vi "Acquire Image.vi"(8 "error in (no error)":errorcluster, 11 "Interface Name":string) -> (0 "error out":errorcluster, 2 "New Image":T1, 3 "Refnum out":T2)   [LabVIEW 2019]
uses:
  <vilib>/userdefined/High Color/IMAQdx.ctl
  <vilib>/vision/Image Controls.llb/IMAQ Image.ctl
  <vilib>/vision/driver/NI_Vision_Acquisition_Software.lvlib
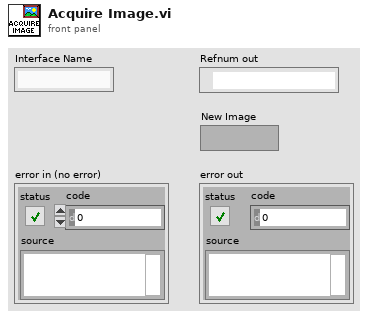
[diagram p1: front panel]
types:
  T1 = typedef "IMAQ Image.ctl" = refnum<image>
  T2 = typedef "IMAQdx.ctl" = refnum<k21>
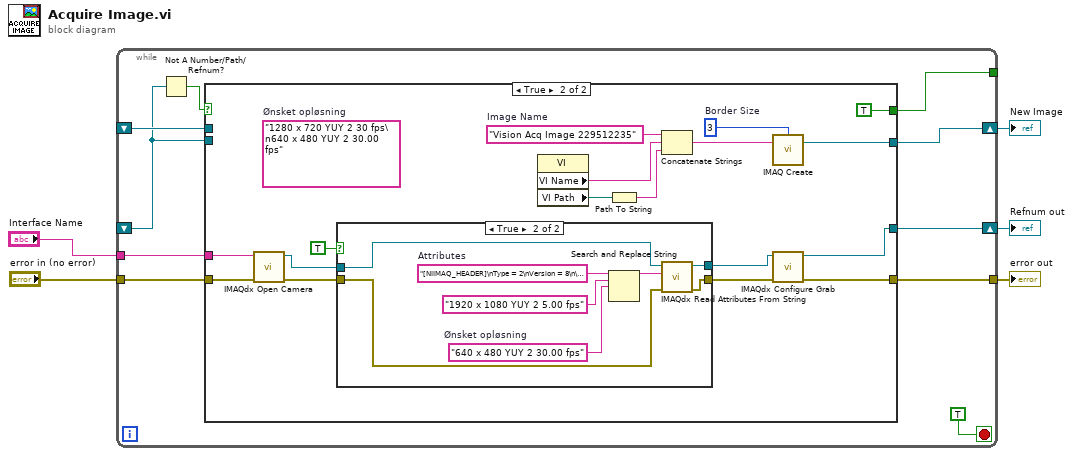
[diagram p0: block diagram]
diagram:
  n1 = while "While Loop_template0" {
    shift-right: [w15] -> w4
    shift-left: _ -> [w8]
    tunnel: [w14] -> w1
    tunnel: "error in (no error)" -> [w13]
    shift-right: [w11] -> w3
    shift-left: _ -> [w10]
    tunnel: "Interface Name" -> [w9]
    tunnel: [w6] -> _
    stop <- TRUE ("_template0") stop-if-true
    n2 = Not A Number/Path/Refnum?(number/path/refnum=w8) -> (NaN/Path/Refnum?=w7:bool)
    n3 = case "Case Structure_template0" shown="True" w7 {
      tunnel: [w18 w34] -> w15
      tunnel: w8 -> [w18 _]
      tunnel: [w17 w33] -> w14
      tunnel: w13 -> [w17 w35]
      tunnel: [w16 w32] -> w11
      tunnel: w10 -> [w16 _]
      tunnel: w9 -> [_ w23]
      tunnel: [_ TRUE] -> w6
      frame False {
      }
      frame True {
        (unwired) "1280 x 720 YUY 2 30 fps\n640 x 480 YUY 2 30.00 fps"  # Ønsket opløsning
        w20 = 3  # Border Size
        w27 = "Vision Acq Image 229512235"  # Image Name
        n4 = call <vilib>:"IMAQdx Open Camera.vi"("error in"=w35, "Session In"=w23) -> ("error out"=w25:errorcluster, "Session Out"=w26:T2)  [unwired: 1 in, 7 out]
        n5 = case shown="True" TRUE ("Init Attributes") {
          tunnel: w26 -> [w37 w45]
          tunnel: w25 -> [w36 w44]
          tunnel: [w37 w43] -> w19
          tunnel: [w36 w42] -> w24
          frame False {
          }
          frame True {
            w38 = "640 x 480 YUY 2 30.00 fps"  # Ønsket opløsning
            w41 = "[NIIMAQ_HEADER]\nType = 2\nVersion = 8\n\n[CAMERA_DATA]\nAcquisitionAttributes::Bayer::Algorithm = \"Bilinear\"\nAcquisitionAttributes::Bayer::GainB = \"1\"\nAcquisitionAttributes::Bayer::GainG = \"1\"\nAcquisitionAttributes::Bayer::GainR = \"1\"\nAcquisitionAttributes::Bayer::Pattern = \"Use hardware value\"\nAcquisitionAttributes::BitsPerPixel = \"Use hardware value\"\nAcquisitionAttributes::HardwareMaximumQueuedBufferCount = \"1000\"\nAcquisitionAttributes::HardwareRequeueBufferListThreshold = \"50\"\nAcquisitionAttributes::IgnoreFirstFrame = \"false\"\nAcquisitionAttributes::ImageDecoderCopyMode = \"Auto\"\nAcquisitionAttributes::OutputImageType = \"Auto\"\nAcquisitionAttributes::OverwriteMode = \"Get Newest\"\nAcquisitionAttributes::PixelSignedness = \"Use hardware value\"\nAcquisitionAttributes::ReceiveTimestampMode = \"None\"\nAcquisitionAttributes::ShiftPixelBits = \"false\"\nAcquisitionAttributes::SwapPixelBytes = \"false\"\nAcquisitionAttributes::Timeout = \"5000\"\nAcquisitionAttributes::VideoMode = \"1920 x 1080 YUY 2 5.00 fps\"\nCameraAttributes::BacklightCompensation::Mode = \"Manual\"\nCameraAttributes::BacklightCompensation::Value = \"0\"\nCameraAttributes::Brightness::Mode = \"Manual\"\nCameraAttributes::Brightness::Value = \"168\"\nCameraAttributes::Contrast::Mode = \"Manual\"\nCameraAttributes::Contrast::Value = \"5\"\nCameraAttributes::Exposure::Mode = \"AutoAperaturePriority\"\nCameraAttributes::Focus::Mode = \"Auto\"\nCameraAttributes::Pan::Mode = \"Manual\"\nCameraAttributes::Pan::Value = \"0\"\nCameraAttributes::PowerLineFrequency::Mode = \"60Hz\"\nCameraAttributes::Saturation::Mode = \"Manual\"\nCameraAttributes::Saturation::Value = \"103\"\nCameraAttributes::Sharpness::Mode = \"Manual\"\nCameraAttributes::Sharpness::Value = \"25\"\nCameraAttributes::Tilt::Mode = \"Manual\"\nCameraAttributes::Tilt::Value = \"0\"\nCameraAttributes::WhiteBalance::Mode = \"Auto\"\nCameraAttributes::Zoom::Mode = \"Manual\"\nCameraAttributes::Zoom::Value = \"0\"\n"  # Attributes
            n6 = Search and Replace String(input string=w41, search string="1920 x 1080 YUY 2 5.00 fps", replace string=w38) -> (result string=w39:string)  [unwired: 5 in, 3 out]
            n7 = call <vilib>:"IMAQdx Read Attributes From String.vi"("error in"=w44, "Attributes String In"=w39, "Session In"=w45) -> ("error out"=w42:errorcluster, "Session Out"=w43:T2)  [unwired: 7 out]
          }
        }
        n8 = property class="VI"() -> ("VI Name"=w30:string, "VI Path"=w31:path)  [unwired: 2 in, 2 out]
        n9 = Path To String(path=w31) -> (string=w29:string)
        n10 = Concatenate Strings(w27, w30, w29) -> (w28:string)
        n11 = call "IMAQ Create"("Border Size"=w20, "Image Name"=w28) -> ("New Image"=w32:T1)  [unwired: 2 in, 2 out]
        n12 = call <vilib>:"IMAQdx Configure Grab.vi"("error in"=w24, "Session In"=w19) -> ("error out"=w33:errorcluster, "Session Out"=w34:T2)  [unwired: 1 in, 7 out]
      }
    }
  }
  "Refnum out" <- w4
  "New Image" <- w3
  "error out" <- w1
